vi "RVC 2-link serial robot Primatic.vi"() -> ()   [LabVIEW 2014]
uses:
  <vilib>/Analysis/Matrix/Datatypes/RealMatrix.ctl
  <vilib>/robotics/Kinematics/Analytical/Initialize Generic Serial Arm.vi
  <vilib>/robotics/Kinematics/Analytical/NI_Robotics_AnalyticKinematics.lvlib
  <vilib>/robotics/Kinematics/Robot/NI_Robotics_Serial Robot Arm.lvclass
  <vilib>/Analysis/Matrix/NI_Matrix.lvlib
panel:
  in  "appended array":dbl[](array[numeric])
  in  "rotation angle (theta)":dbl
  in  "length (a) 2":dbl=0.3 format="%#_13g"
  in  "length (a)":dbl=0.3 format="%#_13g"
  out "transformation":picture
  out "forward kinematics":T1
  out "3D Picture":refnum<vi>(3d-picture)
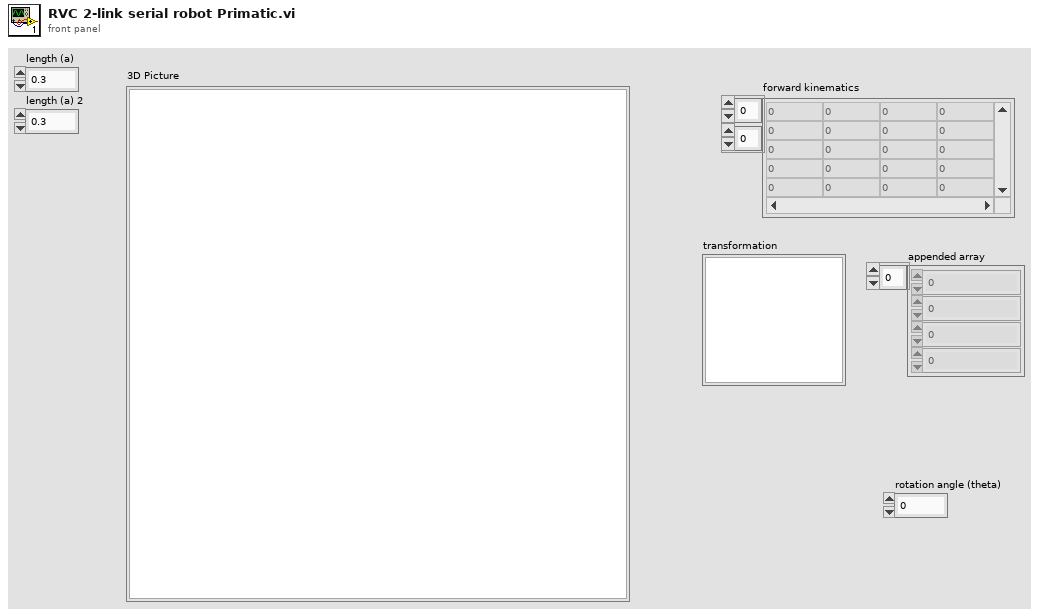
[diagram p1: front panel]
types:
  T1 = typedef "NI_Matrix.lvlib/RealMatrix.ctl" = dbl[][]
  T2 = typedef "DH Kinematic Parameters.ctl" = cluster{"twist angle":dbl, "length":dbl, "rotation angle":dbl, "offset distance":dbl, "joint type":T3, "joint coordinate offset":dbl}
  T3 = typedef "NI_Robotics_Link.lvclass/Joint Type.ctl" = enum16{"Revolute", "Prismatic"}
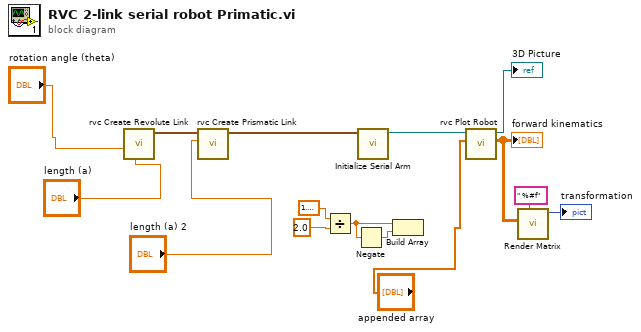
[diagram p0: block diagram]
diagram:
  n1 = call "rvc Create Revolute Link.vi"("length (a)"="length (a)", "twist angle (alpha)"="rotation angle (theta)") -> ("Array"=w8:T2[])  [unwired: 9 in]
  n2 = call "rvc Create Prismatic Link.vi"("length (a)"="length (a) 2", "Array 2"=w8) -> ("Array"=w15:T2[])  [unwired: 9 in]
  n3 = Divide(x=1.5707963267948966, y=2.0) -> (x/y=w10:dbl)
  n4 = Negate(x=w10) -> (-x=w9:dbl)
  n5 = call-poly <vilib>:"Initialize Serial Arm.vi"("kinematic parameters"=w15) -> ("serial arm out"=w14:refnum<class "NI_Robotics_Serial Robot Arm.lvclass">)  [unwired: 9 in, 1 out]
  n6 = Build Array(w10, w9) -> ()  [unwired: 1 out]
  n7 = call "rvc Plot Robot.vi"("joint positions"="appended array", "NI_Robotics_Serial Robot Arm in"=w14) -> ("forward kinematics"=w3:T1, "Scene Object Out"=→"3D Picture":refnum<vi>)  [unwired: 7 in, 1 out]
  "forward kinematics" <- w3
  n8 = call "Render Matrix.vi"("format string"=" %#f", "A"=w3) -> ("picture out"=→"transformation":picture)  [unwired: 9 in]
